vi "usrp_driver_1.vi"() -> ()   [LabVIEW 2021]
doc: "This template is for the Simple NI-USRP Streaming design, a design that shows the basics of streaming data to and from an NI USRP-294x/295x device. Refer to the block diagram for more information about how to use this template."
uses:
  <instrlib>/niUSRP/niUSRP Fetch Rx Data (I16).vi
panel:
  out "coerced IQ rate":dbl=100000.0 format="%#_6p"
  in  "Device Name":refnum<k15>="RIO0"
  out "acquiring":bool caption="Streaming"
  in  "max queue size":i32=100
  out "record time (ms)":u32
  out "write rate (SPS)":dbl format="%#_6p"
  out "# elements in queue":i32
  out "write tdms loop time (ms)":u32
  in  "frequency":dbl=2000000000.0 format="%#_6p"
  in  "sample rate":dbl=50000000.0
  out "get data loop time (ms)":u32 format="%.0p"
  out "error out":errorcluster
  in  "Stop":bool
  # "Overview: Demonstrates the use of the Advanced TDMS and simple streamer functions to write Rx data to a *.tdms file.\nInstructions:\nThis Vi must use Administrator privliges in order to write the data.\nthe USRP sohld be connected via MIXe to the computer (or other direct connection)\nset the params \nRun this VI.\ndue to the way the memory work after some time it can occer that the saveing rate will decrise."
  # "# error NXG style"
  # "Rx Streaming"
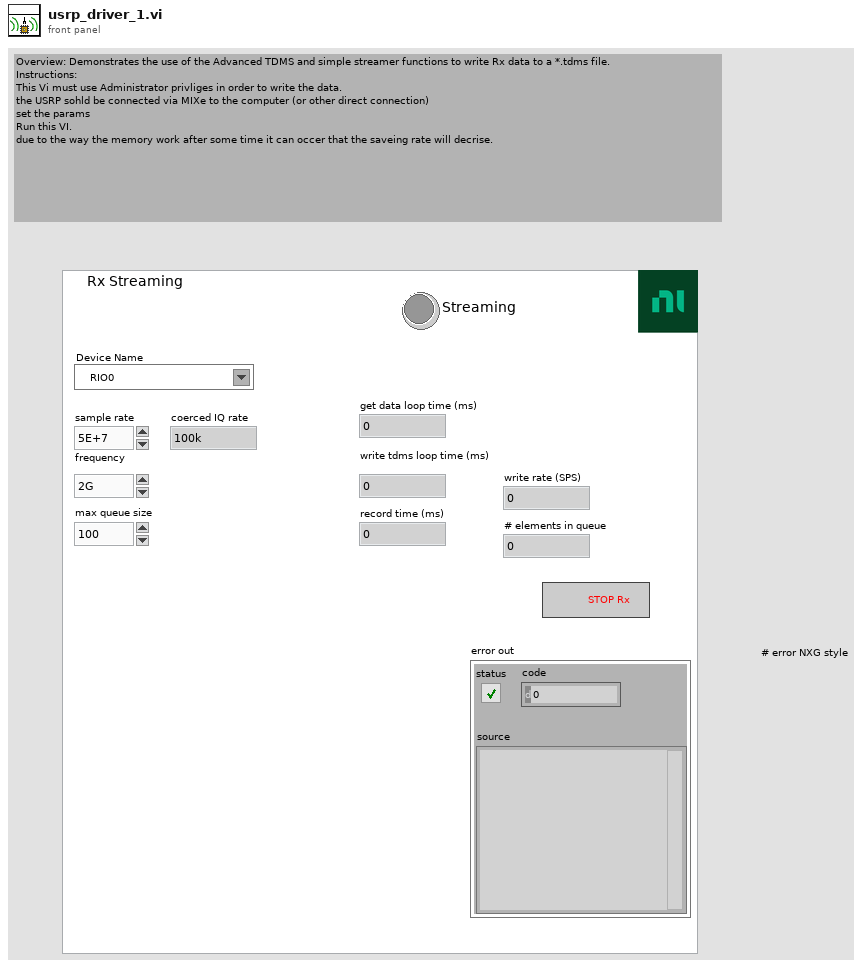
[diagram p1: front panel]
types:
  T1 = enum16{"open", "open or create", "create or replace", "create", "open (read-only)"}
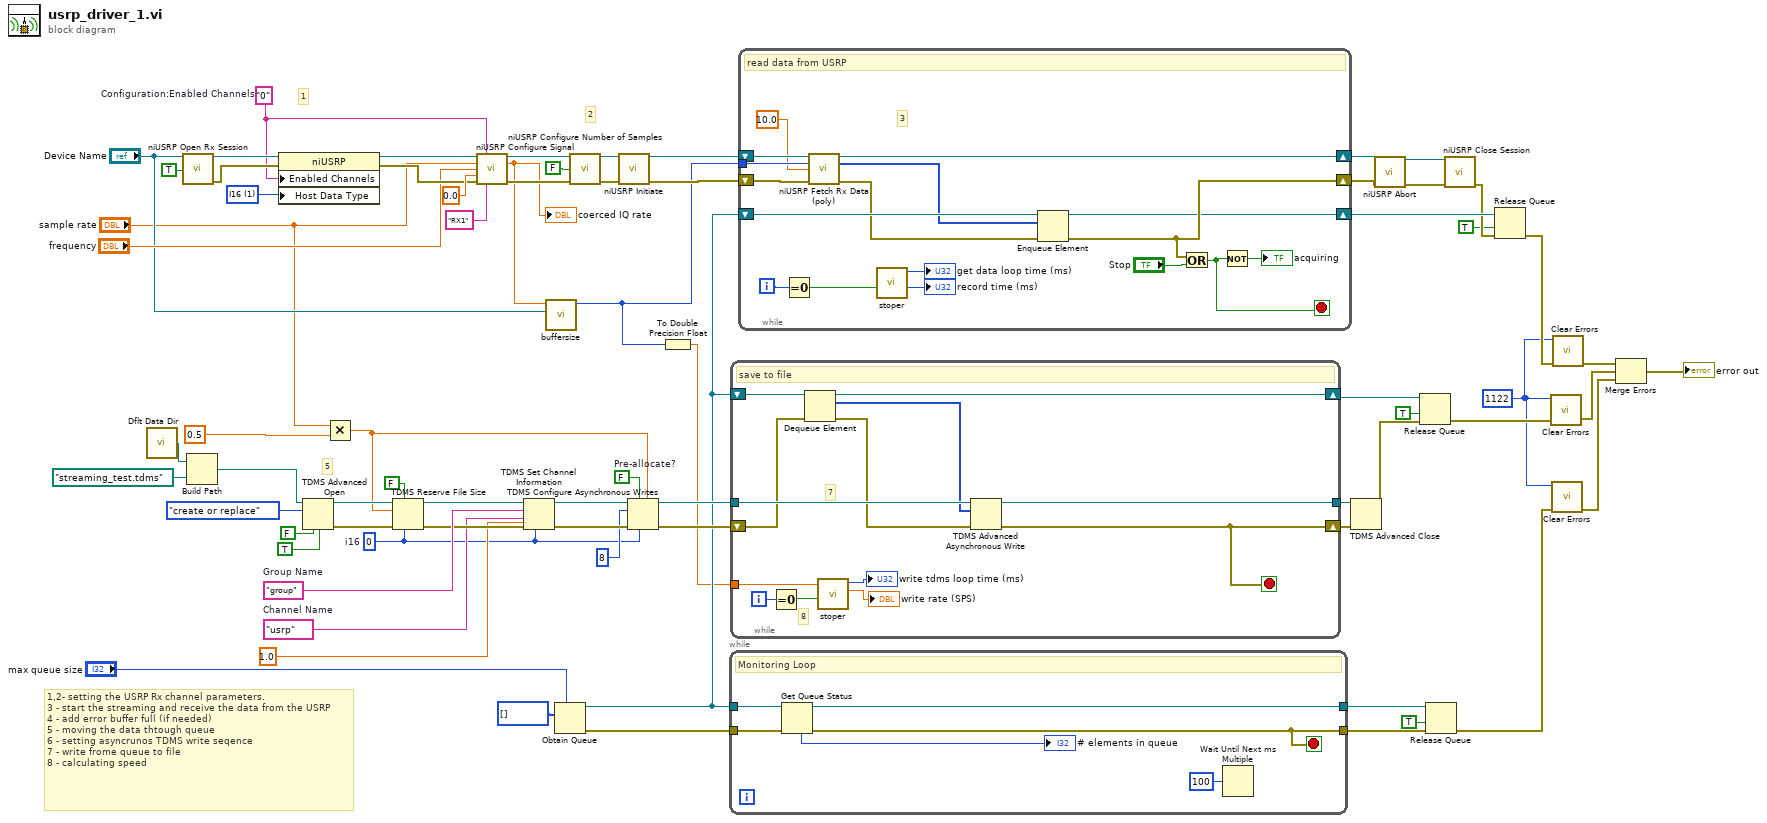
[diagram p0: block diagram]
diagram:
  w10 = 1122 ("specific error code to clear (0: all)")
  w33 = "0"  # Configuration:Enabled Channels
  w45 = 1 items=["CDB", "I16"] ("Configuration:Advanced:Host Data Type")
  w62 = FALSE  # Pre-allocate?
  w52 = i16 0  # i16
  w72 = "group"  # Group Name
  w54 = "usrp"  # Channel Name
  # "2"
  # "1"
  # "1,2- setting the USRP Rx channel parameters.\n3 - start the streaming and receive the data from the USRP\n4 - add error buffer full (if needed)\n5 - moving the data thtough queue   \n6 - setting asyncrunos TDMS write seqence\n7 - write frome queue to file\n8 - calculating speed"
  # "5"
  n1 = call <vilib>:"Dflt Data Dir.vi"() -> ("App:Default Data Directory"=w47:path)
  n2 = call <instrlib>:"niUSRP Open Rx Session.vi"("device names"="Device Name", "reset"=TRUE) -> ("session handle out"=w42:refnum<k15>, "error out"=w43:errorcluster)  [unwired: 12 in]
  n3 = Build Path(base path=w47, name or relative path=path "streaming_test.tdms") -> (appended path=w46:path)
  n4 = property class="niUSRP"(reference=w42, error in=w43, "Enabled Channels"=w33, "Host Data Type"=w45) -> (reference out=w40:refnum<k15>, error out=w38:errorcluster)
  n5 = TDMS Advanced Open(4:TRUE ("enable asynchronous? (T)"), 6:FALSE ("disable buffering? (T)"), 10:T1."create or replace" ("operation (0:open)"), 11:w46) -> (0:w68:errorcluster, 3:w69:refnum<k34>)  [unwired: 1 in, 1 out]
  n6 = Multiply(x="sample rate", y=0.5) -> (x*y=w55:dbl)
  n7 = TDMS Reserve File Size(6:w52, 7:FALSE ("append? (T)"), 8:w68, 10:w55, 11:w69) -> (0:w66:errorcluster, 3:w67:refnum<k34>)
  n8 = call <instrlib>:"niUSRP Configure Signal.vi"("session handle"=w40, "channel list"=w33, "IQ rate"="sample rate", "carrier frequency"="frequency", "gain"=0.0, "error in (no error)"=w38, "active antenna"="RX1") -> ("session handle out"=w36:refnum<k15>, "coerced IQ rate"=w32:dbl, "error out"=w37:errorcluster)  [unwired: 4 in, 2 out]
  "coerced IQ rate" <- w32
  n9 = TDMS Set Channel Information(4:1.0 ("y"), 6:w52, 8:w66, 9:w54, 10:w72, 11:w67) -> (0:w64:errorcluster, 3:w63:refnum<k34>)  [unwired: 1 in]
  n10 = call "buffersize.vi"("Device Name"="Device Name", "coerced IQ rate"=w32) -> ("buffer size"=w3:i64)  [unwired: 9 in]
  n11 = Obtain Queue(max queue size (-1, unlimited)="max queue size", element data type=i16[] [] ("waveform data")) -> (queue out=w14:refnum<queue>, error out=w12:errorcluster)  [unwired: 3 in, 1 out]
  n12 = call <instrlib>:"niUSRP Configure Number of Samples.vi"("session handle"=w36, "number of samples is finite"=FALSE, "error in (no error)"=w37) -> ("session handle out"=w34:refnum<k15>, "error out"=w35:errorcluster)  [unwired: 11 in]
  n13 = call <instrlib>:"niUSRP Initiate.vi"("session handle"=w34, "error in (no error)"=w35) -> ("session handle out"=w30:refnum<k15>, "error out"=w29:errorcluster)  [unwired: 12 in]
  n14 = TDMS Configure Asynchronous Writes(5:w55, 6:w52, 7:w62, 8:w64, 10:u32 8 ("max asynchronous writes (4)"), 11:w63) -> (0:w56:errorcluster, 3:w59:refnum<k34>)  [unwired: 1 in]
  n15 = To Double Precision Float(number=w3) -> (double precision float=w2:dbl)
  n16 = while {
    tunnel: w14 -> [w78]
    tunnel: w12 -> [w76]
    tunnel: [w75] -> w11
    tunnel: [w74] -> w6
    stop <- w75 stop-if-true
    # "Monitoring Loop"
    n17 = Get Queue Status(queue=w78, error in (no error)=w76) -> (queue out=w74:refnum<queue>, error out=w75:errorcluster, # elements in queue=→"# elements in queue":i32)  [unwired: 1 in, 5 out]
    n18 = Wait Until Next ms Multiple(millisecond multiple=u32 100) -> ()  [unwired: 1 out]
  }
  n19 = while {
    tunnel: w59 -> [w90]
    shift-right: [w84] -> w57
    shift-left: w14 -> [w91]
    tunnel: [w88] -> w58
    shift-right: [w89] -> w50
    shift-left: w56 -> [w83]
    tunnel: w2 -> [w80]
    i -> [w86]
    stop <- w89 stop-if-true
    # "8"
    # "7"
    # "save to file"
    n20 = Equal To 0?(x=w86) -> (x = 0?=w81:bool)
    n21 = Dequeue Element(queue=w91, error in (no error)=w83) -> (queue out=w84:refnum<queue>, element=w87:i16[], error out=w82:errorcluster)  [unwired: 1 in, 1 out]
    n22 = call "stoper.vi"("start"=w81, "x mission"=w80) -> ("x rate"=→"write rate (SPS)":dbl, "loop"=→"write tdms loop time (ms)":u32)  [unwired: 7 in, 1 out]
    n23 = TDMS Advanced Asynchronous Write(8:w82, 10:w87, 11:w90) -> (0:w89:errorcluster, 3:w88:refnum<k34>)
  }
  n24 = while {
    tunnel: w3 -> [w106]
    shift-right: [w105] -> w26
    shift-left: w30 -> [w108]
    shift-right: [w104] -> w25
    shift-left: w29 -> [w107]
    shift-right: [w103] -> w22
    shift-left: w14 -> [w102]
    i -> [w92]
    stop <- w93 stop-if-true
    # "3"
    # "read data from USRP"
    n25 = Equal To 0?(x=w92) -> (x = 0?=w94:bool)
    n26 = call-poly <instrlib>:"niUSRP Fetch Rx Data (poly).vi"("session handle"=w108, "number of samples"=w106, "timeout"=10.0, "error in (no error)"=w107) -> ("session handle out"=w105:refnum<k15>, "data"=w96:i16[], "error out"=w95:errorcluster)  [unwired: 8 in, 1 out]
    n27 = call "stoper.vi"("start"=w94) -> ("frome start"=→"record time (ms)":u32, "loop"=→"get data loop time (ms)":u32)  [unwired: 8 in, 1 out]
    n28 = Enqueue Element(queue=w102, element=w96, error in (no error)=w95) -> (queue out=w103:refnum<queue>, error out=w104:errorcluster)  [unwired: 1 in, 1 out]
    n29 = Or(x=w104, y="Stop") -> (x .or. y?=w93:bool)
    n30 = Not(x=w93) -> (.not. x?=→"acquiring":bool)
  }
  n31 = TDMS Advanced Close(8:w50, 11:w58) -> (0:w23:errorcluster)  [unwired: 2 in, 1 out]
  n32 = call <instrlib>:"niUSRP Abort.vi"("session handle"=w26, "error in (no error)"=w25) -> ("session handle out"=w27:refnum<k15>, "error out"=w28:errorcluster)  [unwired: 12 in]
  n33 = Release Queue(queue=w57, force destroy? (F)=TRUE, error in (no error)=w23) -> (error out=w15:errorcluster)  [unwired: 2 out]
  n34 = Release Queue(queue=w6, force destroy? (F)=TRUE, error in (no error)=w11) -> (error out=w8:errorcluster)  [unwired: 2 out]
  n35 = call <instrlib>:"niUSRP Close Session.vi"("session handle"=w27, "error in (no error)"=w28) -> ("error out"=w21:errorcluster)  [unwired: 13 in]
  n36 = Release Queue(queue=w22, force destroy? (F)=TRUE, error in (no error)=w21) -> (error out=w16:errorcluster)  [unwired: 2 out]
  n37 = call <vilib>:"Clear Errors.vi"("error in (no error)"=w15, "specific error code to clear (0: all)"=w10) -> ("error out"=w9:errorcluster)  [unwired: 4 in, 1 out]
  n38 = call <vilib>:"Clear Errors.vi"("error in (no error)"=w8, "specific error code to clear (0: all)"=w10) -> ("error out"=w7:errorcluster)  [unwired: 4 in, 1 out]
  n39 = call <vilib>:"Clear Errors.vi"("error in (no error)"=w16, "specific error code to clear (0: all)"=w10) -> ("error out"=w17:errorcluster)  [unwired: 4 in, 1 out]
  n40 = Merge Errors(w17, w9, w7) -> (→"error out":errorcluster)
